vi "OE1022D_Configure Dynamic Reserve.vi"(0 "VISA resource name":refnum<visa-resource-name>, 1 "OE1022D A/B":u8(ring) items=["Channel A", "Channel B"], 2 "Reserve":u8(ring) items=["Low", "Normal", "High"], 5 "error in (no error)":errorcluster) -> (14 "VISA resource name out":refnum<visa-resource-name>, 15 "发送命令":string, 19 "error out":errorcluster)   [LabVIEW 2021]
doc: "Configures the reference source and the internal oscillator."
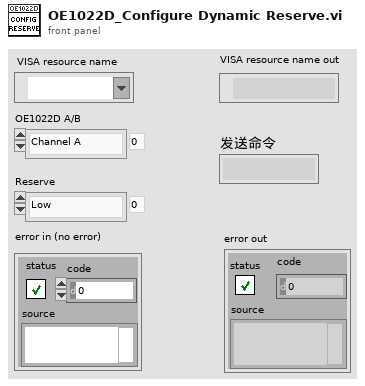
[diagram p1: front panel]
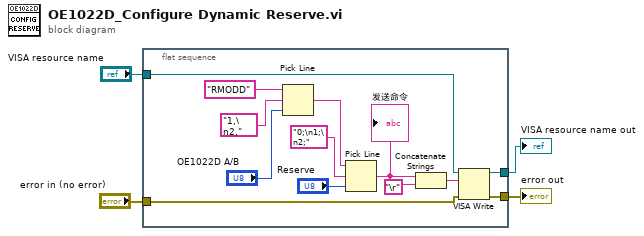
[diagram p0: block diagram]
diagram:
  n1 = flat-sequence {
    tunnel: "error in (no error)" -> [w16]
    tunnel: "VISA resource name" -> [w17]
    tunnel: [w15] -> w4
    tunnel: [w14] -> w3
    frame #0 {
      n2 = Pick Line(string ("")="RMODD", multi-line string="1,\n2,", line index="OE1022D A/B") -> (output string=w7:string)
      n3 = Pick Line(string ("")=w7, multi-line string="0;\n1;\n2;", line index="Reserve") -> (output string=w6:string)
      "发送命令" <- w6
      n4 = Concatenate Strings(w6, "\r" ("字符串")) -> (w5:string)
      n5 = VISA Write(VISA resource name=w17, write buffer=w5, error in (no error)=w16) -> (VISA resource name out=w15:refnum<visa-resource-name>, error out=w14:errorcluster)  [unwired: 1 out]
    }
  }
  "error out" <- w3
  "VISA resource name out" <- w4
